vi "Read Gantry Controller A3200.vi"(8 "error in (no error)":errorcluster, 11 "Gantry in":refnum<class "Gantry.lvclass">) -> (0 "error out":errorcluster, 2 "A3200 controller out":refnum<k24>, 3 "Gantry out":refnum<class "Gantry.lvclass">)   [LabVIEW 2024, in "Gantry.lvclass"]
uses:
  Gantry.lvclass
  Gantry.lvclass/Gantry.ctl
  C:/Users/cfang/Desktop/nebraska-silicon-lab/pixel-gantry-control/Gantry/A3200/Bin/Aerotech.A3200.dll
  A3200/Bin/Aerotech.A3200.dll
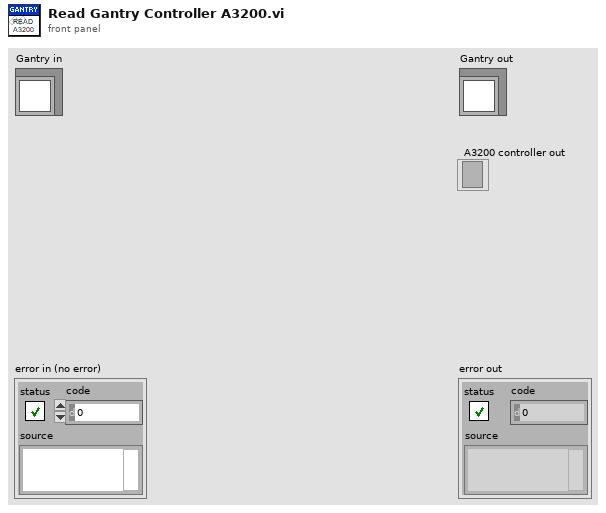
[diagram p1: front panel]
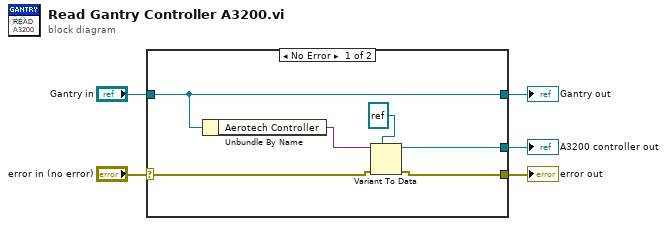
[diagram p0: block diagram]
diagram:
  n1 = case shown="No Error" "error in (no error)" {
    selector: "error in (no error)" -> [w8 w13]
    tunnel: [w7 w13] -> w4
    tunnel: [w11 w12] -> w2
    tunnel: "Gantry in" -> [w11 w12]
    tunnel: [w6 _] -> w1
    frame No Error {
      n2 = Unbundle By Name(w11) -> ("Aerotech Controller"=w10:variant)
      n3 = Variant To Data(error in=w8, type=refnum<k24> refnum ("controller out"), Variant=w10) -> (data=w6:refnum<k24>, error out=w7:errorcluster)
    }
    frame Error {
    }
  }
  "error out" <- w4
  "Gantry out" <- w2
  "A3200 controller out" <- w1
